vi "colour.get.vi"(11 "Game Componants in":refnum<class "Game Componants.lvclass">) -> (2 "Componant Colour":u32(colorbox))   [LabVIEW 2020, in "Game Componants.lvclass"]
uses:
  Game Componants.lvclass
  Game Componants.lvclass/Game Componants.ctl
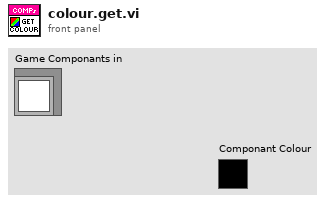
[diagram p1: front panel]
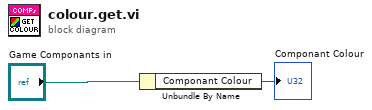
[diagram p0: block diagram]
diagram:
  n1 = Unbundle By Name("Game Componants in") -> ("Componant Colour"=→"Componant Colour":u32)
